vi "SendNotifiction.vi"(8 "error in (no error)":errorcluster, 11 "VIActivation in":refnum<class "VIActivation.lvclass">) -> (0 "error out":errorcluster, 3 "VIActivation out":refnum<class "VIActivation.lvclass">)   [LabVIEW 2021]
uses:
  VIActivation.lvclass
  VIActivation.lvclass/VIActivation.ctl
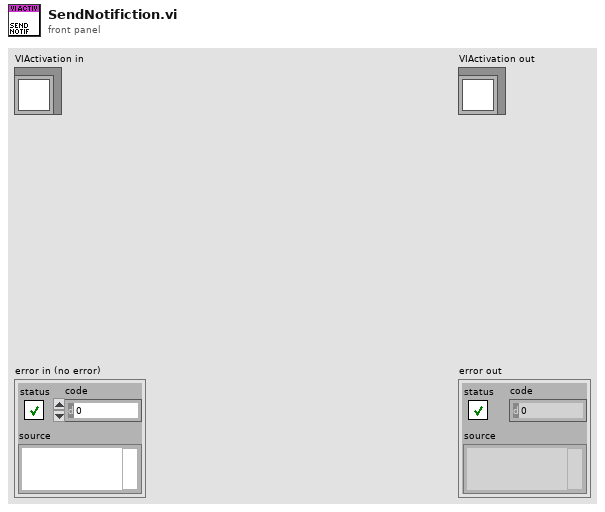
[diagram p1: front panel]
types:
  T1 = typedef "VIActivation.lvlib/VIActivation.lvclass/data.ctl" = cluster{"VIActivation":refnum<user-event>, "VIDesactivation":refnum<user-event>, "notifier":refnum<notifier>, "CloseEvent":refnum<user-event>}
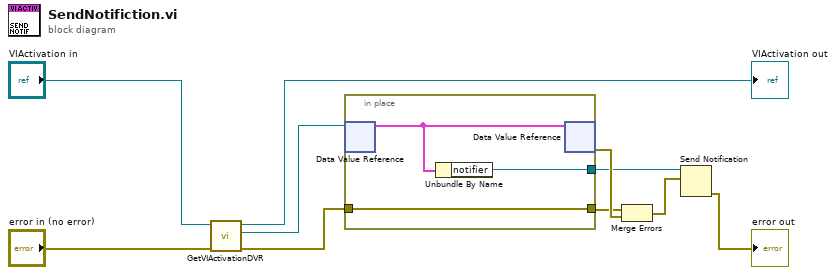
[diagram p0: block diagram]
diagram:
  n1 = call "GetVIActivationDVR.vi"("error in (no error)"="error in (no error)", "VIActivation in"="VIActivation in") -> ("error out"=w3:errorcluster, "DVR"=w4:refnum<data-value>, "VIActivation out"=→"VIActivation out":refnum<class "VIActivation.lvclass">)  [unwired: 7 in]
  n2 = in-place {
    in-place-border: w3 -> [w13]
    in-place-border: [w13] -> w5
    in-place-border: [w11] -> w2
    n3 = in-place-dvr #1(w4) -> (w12:T1)  [unwired: 1 out]
    n4 = Unbundle By Name(w12) -> ("notifier"=w11:refnum<notifier>)
    n5 = in-place-dvr #1(w12) -> (w6:errorcluster)  [unwired: 1 out]
  }
  n6 = Merge Errors(w5, w6) -> (w1:errorcluster)
  n7 = Send Notification(notification=w1, notifier=w2) -> (error out=→"error out":errorcluster)  [unwired: 1 in, 1 out]
